vi "Query.vi"(6 "error":errorcluster, 8 "Quantity":string(combo), 9 "VISA resource name":refnum<visa-resource-name>) -> (0 "error out":errorcluster, 2 "Value":dbl format="%_4f", 3 "VISA resource name out":refnum<visa-resource-name>, 5 "Response":string)   [LabVIEW 2018, in "BigSkyControl.lvlib"]
uses:
  BigSkyControl.lvlib
panel:
  out "Read return count":u32
  in  "byte count":u32=1024
  out "Write return count":u32
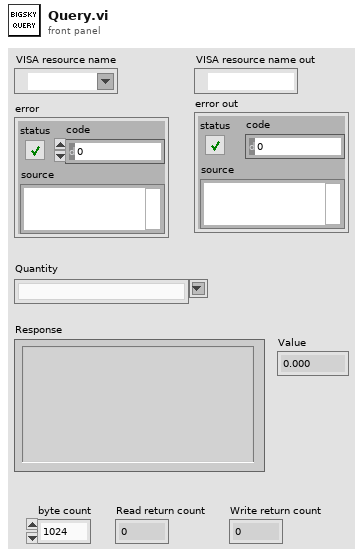
[diagram p1: front panel]
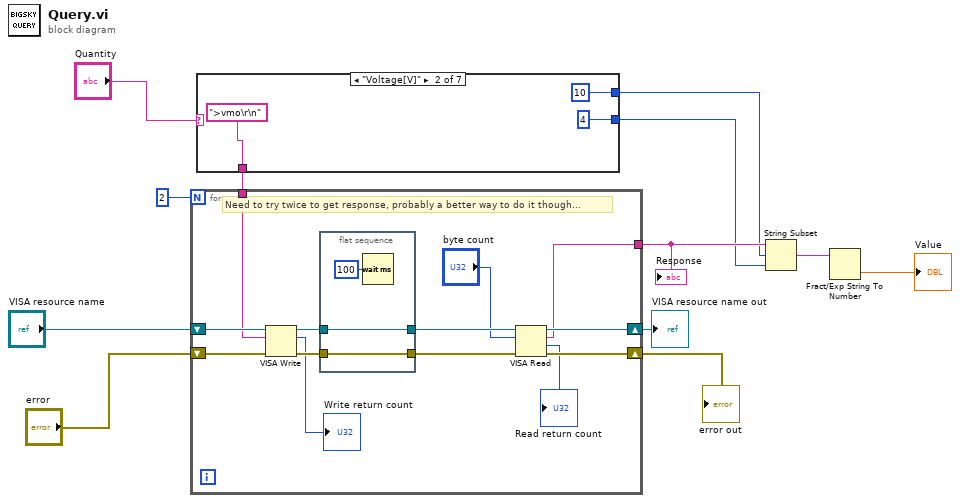
[diagram p0: block diagram]
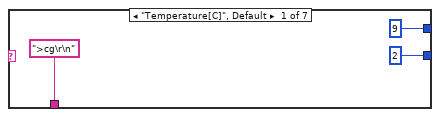
[diagram p2: hidden frame]
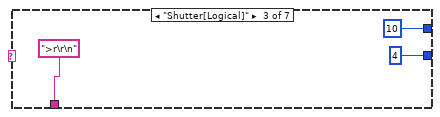
[diagram p3: hidden frame]
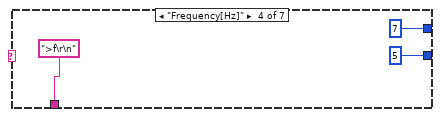
[diagram p4: hidden frame]
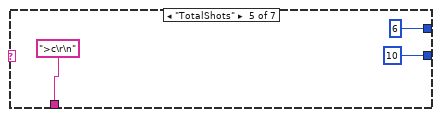
[diagram p5: hidden frame]
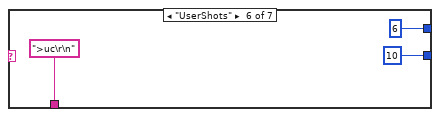
[diagram p6: hidden frame]
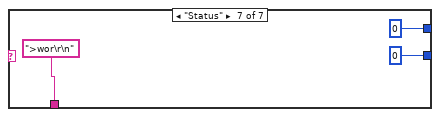
[diagram p7: hidden frame]
diagram:
  n1 = case shown="\"Voltage[V]\"" "Quantity" {
    tunnel: [">cg\r\n" ("write buffer") ">vmo\r\n" ("write buffer") ">r\r\n" ("write buffer") ">f\r\n" ("write buffer") ">c\r\n" ("write buffer") ">uc\r\n" ("write buffer") ">wor\r\n" ("write buffer")] -> w5
    tunnel: [9 ("offset (0)") 10 ("offset (0)") 10 ("offset (0)") 7 ("offset (0)") 6 ("offset (0)") 6 ("offset (0)") 0 ("offset (0)")] -> w4
    tunnel: [2 ("length (rest)") 4 ("length (rest)") 4 ("length (rest)") 5 ("length (rest)") 10 ("length (rest)") 10 ("length (rest)") 0 ("length (rest)")] -> w3
    frame "Temperature[C]", Default {
    }
    frame "Voltage[V]" {
    }
    frame "Shutter[Logical]" {
    }
    frame "Frequency[Hz]" {
    }
    frame "TotalShots" {
    }
    frame "UserShots" {
    }
    frame "Status" {
    }
  }
  n2 = for {
    N: 2 -> [_]
    shift-right: [w45] -> w9
    shift-left: "VISA resource name" -> [w44]
    shift-right: [w46] -> w8
    shift-left: "error" -> [w43]
    tunnel: [w35] -> w7
    tunnel: w5 -> [w34]
    # "Need to try twice to get response, probably a better way to do it though..."
    n3 = VISA Write(VISA resource name=w44, write buffer=w34, error in (no error)=w43) -> (VISA resource name out=w41:refnum<visa-resource-name>, return count=→"Write return count":u32, error out=w42:errorcluster)
    n4 = flat-sequence {
      tunnel: w42 -> [w49]
      tunnel: [w49] -> w39
      tunnel: w41 -> [w48]
      tunnel: [w48] -> w40
      frame #0 {
        n5 = Wait (ms)(milliseconds to wait=u32 100) -> ()  [unwired: 1 out]
      }
    }
    n6 = VISA Read(VISA resource name=w40, byte count="byte count", error in (no error)=w39) -> (VISA resource name out=w45:refnum<visa-resource-name>, read buffer=w35:string, return count=→"Read return count":u32, error out=w46:errorcluster)
  }
  "Response" <- w7
  "VISA resource name out" <- w9
  "error out" <- w8
  n7 = String Subset(string=w7, offset (0)=w4, length (rest)=w3) -> (substring=w6:string)
  n8 = Fract/Exp String To Number(string=w6) -> (number=→"Value":dbl)  [unwired: 3 in, 1 out]
